vi "Meas Result Generate TWM Digitizer Correction - Generate Files.vi"(8 "error in (no error)":errorcluster, 10 "correction data":T1, 11 "correction root file":path) -> (0 "error out":errorcluster)   [LabVIEW 2020]
uses:
  Meas Results TWM Digitizer Correction Data.ctl
  Meas Results Correction Structuring Mode.ctl
  other/infolib/String.vi
  other/infolib/I64.vi
  other/infolib/2D EXT.vi
  other/infolib/1D EXT.vi
  other/infolib/1D String.vi
  other/infolib/1D I64.vi
  other/infolib/infolib.lvlib
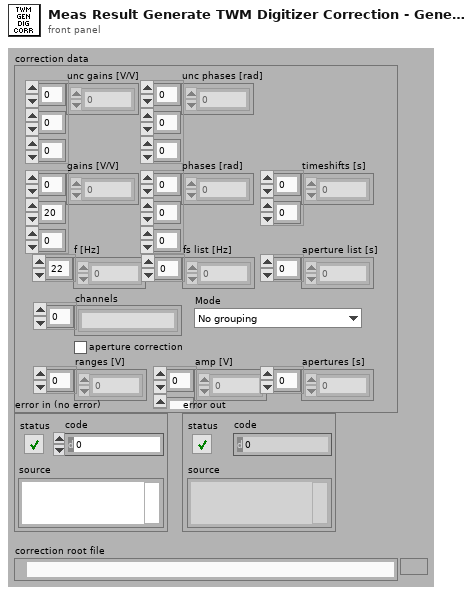
[diagram p1: front panel]
types:
  T1 = typedef "Meas Results TWM Digitizer Correction Data.ctl" = cluster{"gains [V/V]":dbl[][][], "phases [rad]":dbl[][][], "timeshifts [s]":dbl[][], "f [Hz]":dbl[], "fs list [Hz]":dbl[], "aperture list [s]":dbl[], "channels":string[], "Mode":T2, "aperture correction":bool, "ranges [V]":dbl[], "amp [V]":dbl[][], "apertures [s]":dbl[], "unc gains [V/V]":dbl[][][], "unc phases [rad]":dbl[][][]}
  T2 = typedef "Meas Results Correction Structuring Mode.ctl" = enum16{"No grouping", "Group by apertures (3458A)", "Group by fs (generic digitizer)"}
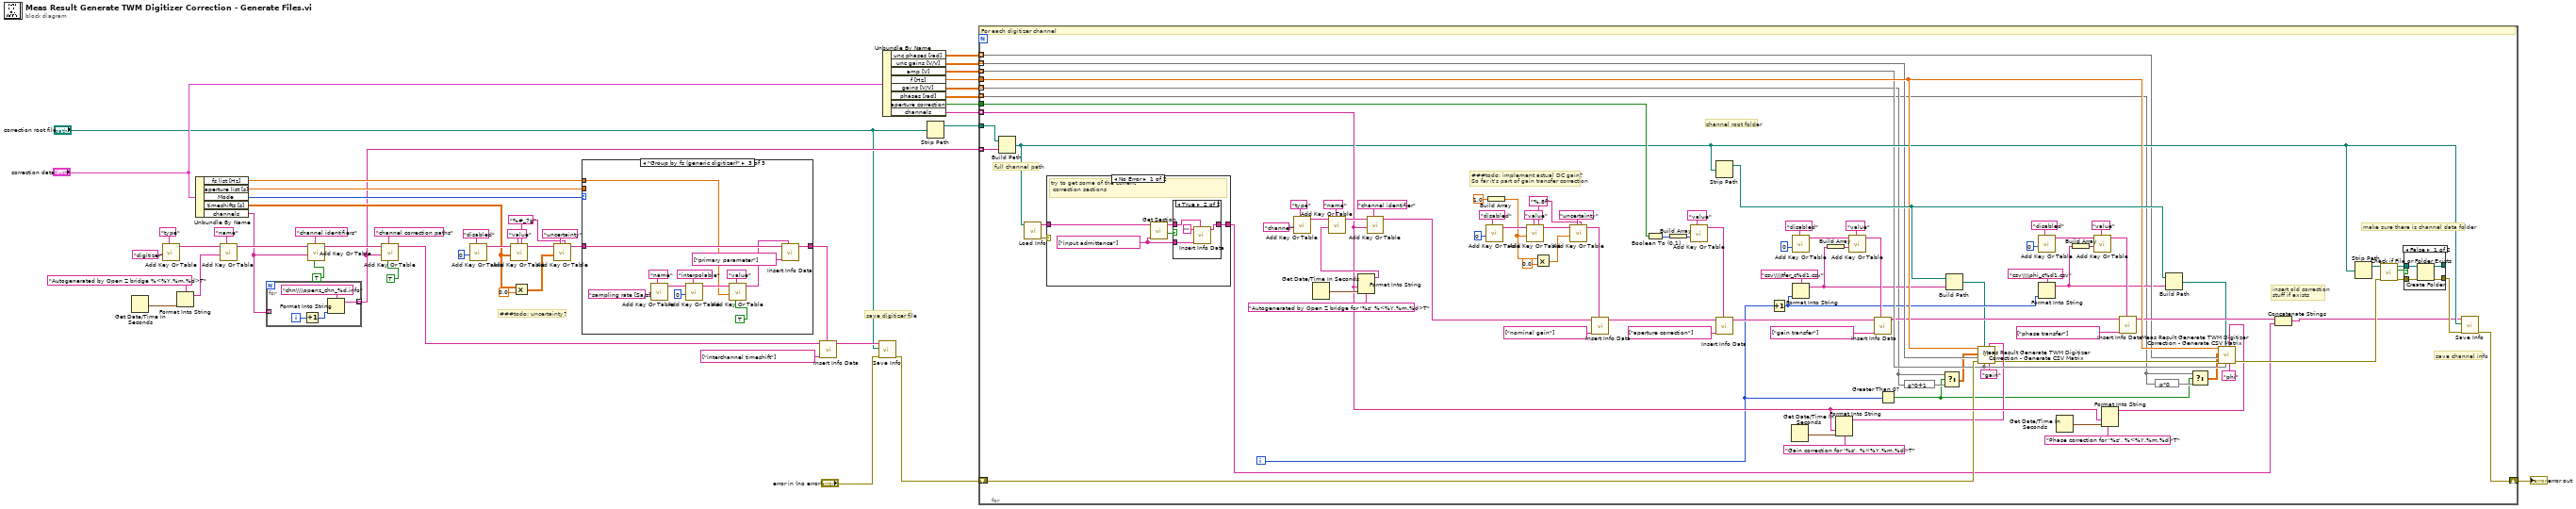
[diagram p0: block diagram]
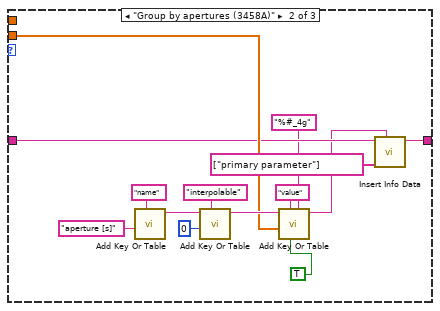
[diagram p6: hidden frame]
diagram:
  w8 = "%#_7g" ("format string (%_20f)")
  # "save digitizer file"
  # "###todo: uncertainty?"
  n1 = Get Date/Time In Seconds() -> (seconds since 1Jan1904=w42:timestamp)
  n2 = call-poly "Add Key Or Table.vi"("key description"="type", "string"="digitizer") -> ("info data out"=w44:string)  [unwired: 8 in, 1 out]
  n3 = Format Into String(format string="Autogenerated by Open Z bridge %<%Y.%m.%d>T", w42) -> (resulting string=w41:string)  [unwired: 2 in, 1 out]
  n4 = Unbundle By Name("correction data") -> ("fs list [Hz]"=w23:dbl[], "aperture list [s]"=w24:dbl[], "Mode"=w25:T2, "timeshifts [s]"=w29:dbl[][], "channels"=w36:string[])
  n5 = call-poly "Add Key Or Table.vi"("key description"="name", "string"=w41, "info data"=w44) -> ("info data out"=w39:string)  [unwired: 7 in, 1 out]
  n6 = for {
    tunnel: w36 -> [_] mode=indexing
    tunnel: [w50] -> w19 mode=indexing
    i -> [w49]
    n7 = Increment(x=w49) -> (x+1=w48:i32)
    n8 = Format Into String(format string="chn\\\\openz_chn_%d.info", w48) -> (resulting string=w50:string)  [unwired: 2 in, 1 out]
  }
  n9 = call-poly "Add Key Or Table.vi"("collumn vector (F)"=TRUE ("column vector (F)"), "key description"="channel identifiers", "string"=w36, "info data"=w39) -> ("info data out"=w37:string)  [unwired: 6 in, 1 out]
  n10 = call-poly "Add Key Or Table.vi"("collumn vector (F)"=TRUE ("column vector (F)"), "key description"="channel correction paths", "string"=w19, "info data"=w37) -> ("info data out"=w21:string)  [unwired: 6 in, 1 out]
  n11 = call-poly "Add Key Or Table.vi"("key description"="disabled", "numeric"=i64 0) -> ("info data out"=w32:string)  [unwired: 8 in, 1 out]
  n12 = call-poly "Add Key Or Table.vi"("format string (%.;%#_20f)"=w8, "key description"="value", "numeric"=w29, "info data"=w32) -> ("info data out"=w30:string)  [unwired: 6 in, 1 out]
  n13 = Multiply(x=w29, y=0.0) -> (x*y=w28:dbl[][])
  n14 = call-poly "Add Key Or Table.vi"("format string (%.;%#_20f)"=w8, "key description"="uncertainty", "numeric"=w28, "info data"=w30) -> ("info data out"=w26:string)  [unwired: 6 in, 1 out]
  n15 = case shown="\"Group by fs (generic digitizer)\"" w25 {
    tunnel: w26 -> [w52 w58 w72]
    tunnel: w24 -> [_ w59 _]
    tunnel: [w52 w55 w69] -> w22
    tunnel: w23 -> [_ _ w68]
    frame "No grouping", Default {
    }
    frame "Group by apertures (3458A)" {
      n16 = call-poly "Add Key Or Table.vi"("key description"="name", "string"="aperture [s]") -> ("info data out"=w63:string)  [unwired: 8 in, 1 out]
      n17 = call-poly "Add Key Or Table.vi"("key description"="interpolable", "numeric"=i64 0, "info data"=w63) -> ("info data out"=w60:string)  [unwired: 7 in, 1 out]
      n18 = call-poly "Add Key Or Table.vi"("format string (%.;%#_20f)"="%#_4g" ("format string (%_20f)"), "collumn vector (F)"=TRUE ("column vector (F)"), "key description"="value", "numeric"=w59, "info data"=w60) -> ("info data out"=w57:string)  [unwired: 5 in, 1 out]
      n19 = call "Insert Info Data.vi"("info data to insert"=w57, "sections"=string[] ["primary parameter"], "info data"=w58) -> ("info data out"=w55:string)  [unwired: 7 in, 1 out]
    }
    frame "Group by fs (generic digitizer)" {
      n20 = call-poly "Add Key Or Table.vi"("key description"="name", "string"="sampling rate [Sa/s]") -> ("info data out"=w76:string)  [unwired: 8 in, 1 out]
      n21 = call-poly "Add Key Or Table.vi"("key description"="interpolable", "numeric"=i64 0, "info data"=w76) -> ("info data out"=w73:string)  [unwired: 7 in, 1 out]
      n22 = call-poly "Add Key Or Table.vi"("collumn vector (F)"=TRUE ("column vector (F)"), "key description"="value", "numeric"=w68, "info data"=w73) -> ("info data out"=w71:string)  [unwired: 6 in, 1 out]
      n23 = call "Insert Info Data.vi"("info data to insert"=w71, "sections"=string[] ["primary parameter"], "info data"=w72) -> ("info data out"=w69:string)  [unwired: 7 in, 1 out]
    }
  }
  n24 = call "Insert Info Data.vi"("info data to insert"=w22, "sections"=string[] ["interchannel timeshift"], "info data"=w21) -> ("info data out"=w15:string)  [unwired: 7 in, 1 out]
  n25 = call "Save Info.vi"("error in"="error in (no error)", "filename"="correction root file", "info data"=w15) -> ("error out"=w13:errorcluster)  [unwired: 8 in]
  n26 = Unbundle By Name("correction data") -> ("unc phases [rad]"=w3:dbl[][][], "unc gains [V/V]"=w4:dbl[][][], "amp [V]"=w5:dbl[][], "f [Hz]"=w9:dbl[], "gains [V/V]"=w7:dbl[][][], "phases [rad]"=w6:dbl[][][], "aperture correction"=w16:bool, "channels"=w17:string[])
  n27 = Strip Path(path="correction root file") -> (stripped path=w12:path)  [unwired: 1 out]
  n28 = for {
    tunnel: w19 -> [w171] mode=indexing
    tunnel: w12 -> [w170]
    tunnel: w17 -> [w133] mode=indexing
    tunnel: w16 -> [w142]
    shift-right: [w135] -> w10
    shift-left: w13 -> [w131]
    tunnel: w6 -> [w81] mode=indexing
    tunnel: w9 -> [w132]
    tunnel: w7 -> [w84] mode=indexing
    tunnel: w5 -> [w121] mode=indexing
    tunnel: w4 -> [w120] mode=indexing
    tunnel: w3 -> [w119] mode=indexing
    i -> [w86]
    w128 = "%.8f" ("format string (%_20f)")
    # "insert old correction\nstuff if exists"
    # "full channel path"
    # "channel root folder"
    # "make sure there is channel data folder"
    # "save channel info"
    # "###todo: implement actual DC gain?\nSo far it's part of gain transfer correction"
    # "For each digitizer channel"
    n29 = Build Path(base path=w170, name or relative path=w171) -> (appended path=w127:path)
    n30 = call "Load Info.vi"("filename"=w127) -> ("error out"=w126:errorcluster, "info data"=w125:string)  [unwired: 9 in]
    n31 = case shown="No Error" w126 {
      tunnel: w125 -> [w176 _]
      tunnel: [w173 _] -> w122
      frame No Error {
        w172 = string[] ["input admittance"] ("sections")
        # "try to get some of the current\n correction sections"
        n32 = call "Get Section.vi"("sections"=w172, "info data"=w176) -> ("exist"=w175:bool, "section part"=w174:string)  [unwired: 7 in, 1 out]
        n33 = case shown="True" w175 {
          tunnel: w174 -> [_ w178]
          tunnel: w172 -> [_ w180]
          tunnel: [_ w179] -> w173
          frame False {
          }
          frame True {
            n34 = call "Insert Info Data.vi"("info data to insert"=w178, "sections"=w180, "info data"="") -> ("info data out"=w179:string)  [unwired: 7 in, 1 out]
          }
        }
      }
      frame Error {
      }
    }
    n35 = call-poly "Add Key Or Table.vi"("key description"="type", "string"="channel") -> ("info data out"=w167:string)  [unwired: 8 in, 1 out]
    n36 = Get Date/Time In Seconds() -> (seconds since 1Jan1904=w163:timestamp)
    n37 = Format Into String(format string="Autogenerated by Open Z bridge for '%s' %<%Y.%m.%d>T", w133, w163) -> (resulting string=w161:string)  [unwired: 2 in, 1 out]
    n38 = call-poly "Add Key Or Table.vi"("key description"="name", "string"=w161, "info data"=w167) -> ("info data out"=w169:string)  [unwired: 7 in, 1 out]
    n39 = call-poly "Add Key Or Table.vi"("key description"="channel identifier", "string"=w133, "info data"=w169) -> ("info data out"=w149:string)  [unwired: 7 in, 1 out]
    n40 = call-poly "Add Key Or Table.vi"("key description"="disabled", "numeric"=i64 0) -> ("info data out"=w158:string)  [unwired: 8 in, 1 out]
    n41 = Build Array(1.0) -> (w152:dbl[])
    n42 = call-poly "Add Key Or Table.vi"("format string (%.;%#_20f)"=w128, "key description"="value", "numeric"=w152, "info data"=w158) -> ("info data out"=w160:string)  [unwired: 6 in, 1 out]
    n43 = Multiply(x=w152, y=0.0) -> (x*y=w153:dbl[])
    n44 = call-poly "Add Key Or Table.vi"("format string (%.;%#_20f)"=w128, "key description"="uncertainty", "numeric"=w153, "info data"=w160) -> ("info data out"=w150:string)  [unwired: 6 in, 1 out]
    n45 = call "Insert Info Data.vi"("info data to insert"=w150, "sections"=string[] ["nominal gain"], "info data"=w149) -> ("info data out"=w145:string)  [unwired: 7 in, 1 out]
    n46 = Boolean To (0,1)(Boolean=w142) -> (0, 1=w143:i16)
    n47 = Build Array(w143) -> (w129:i16[])
    n48 = call-poly "Add Key Or Table.vi"("key description"="value", "numeric"=w129) -> ("info data out"=w144:string)  [unwired: 8 in, 1 out]
    n49 = Strip Path(path=w127) -> (stripped path=w134:path)  [unwired: 1 out]
    n50 = call "Insert Info Data.vi"("info data to insert"=w144, "sections"=string[] ["aperture correction"], "info data"=w145) -> ("info data out"=w141:string)  [unwired: 7 in, 1 out]
    n51 = Increment(x=w86) -> (x+1=w101:i32)
    n52 = Get Date/Time In Seconds() -> (seconds since 1Jan1904=w98:timestamp)
    n53 = call-poly "Add Key Or Table.vi"("key description"="disabled", "numeric"=i64 0) -> ("info data out"=w115:string)  [unwired: 8 in, 1 out]
    n54 = Format Into String(format string="csv\\\\tfer_c%d1.csv", w101) -> (resulting string=w100:string)  [unwired: 2 in, 1 out]
    n55 = Build Array(w100) -> (w111:string[])
    n56 = Format Into String(format string="Gain correction for '%s', %<%Y.%m.%d>T", w133, w98) -> (resulting string=w96:string)  [unwired: 2 in, 1 out]
    n57 = call-poly "Add Key Or Table.vi"("key description"="value", "string"=w111, "info data"=w115) -> ("info data out"=w113:string)  [unwired: 7 in, 1 out]
    n58 = call "Insert Info Data.vi"("info data to insert"=w113, "sections"=string[] ["gain transfer"], "info data"=w141) -> ("info data out"=w102:string)  [unwired: 7 in, 1 out]
    n59 = Greater Than 0?(x=w86) -> (x > 0?=w80:bool)
    n60 = expression code="g*0+1"(w84) -> (w85:dbl[][])
    n61 = Select(t=w84, s=w80, f=w85) -> (s? t:f=w87:dbl[][])
    n62 = Build Path(base path=w134, name or relative path=w100) -> (appended path=w99:path)
    n63 = call "Meas Result Generate TWM Digitizer Correction - Generate CSV Matrix.vi"("header"="gain", "comment"=w96, "amp [V]"=w121, "CSV path"=w99, "error in (no error)"=w131, "uncertainty"=w120, "data"=w87, "f [Hz]"=w132) -> ("error out"=w91:errorcluster)  [unwired: 3 in]
    n64 = call-poly "Add Key Or Table.vi"("key description"="disabled", "numeric"=i64 0) -> ("info data out"=w106:string)  [unwired: 8 in, 1 out]
    n65 = Format Into String(format string="csv\\\\phi_c%d1.csv", w101) -> (resulting string=w92:string)  [unwired: 2 in, 1 out]
    n66 = Get Date/Time In Seconds() -> (seconds since 1Jan1904=w93:timestamp)
    n67 = Build Array(w92) -> (w110:string[])
    n68 = call-poly "Add Key Or Table.vi"("key description"="value", "string"=w110, "info data"=w106) -> ("info data out"=w108:string)  [unwired: 7 in, 1 out]
    n69 = Format Into String(format string="Phase correction for '%s', %<%Y.%m.%d>T", w133, w93) -> (resulting string=w95:string)  [unwired: 2 in, 1 out]
    n70 = call "Insert Info Data.vi"("info data to insert"=w108, "sections"=string[] ["phase transfer"], "info data"=w102) -> ("info data out"=w124:string)  [unwired: 7 in, 1 out]
    n71 = expression code="p*0"(w81) -> (w83:dbl[][])
    n72 = Build Path(base path=w134, name or relative path=w92) -> (appended path=w90:path)
    n73 = Select(t=w81, s=w80, f=w83) -> (s? t:f=w82:dbl[][])
    n74 = call "Meas Result Generate TWM Digitizer Correction - Generate CSV Matrix.vi"("header"="phi", "comment"=w95, "amp [V]"=w121, "CSV path"=w90, "error in (no error)"=w91, "uncertainty"=w119, "data"=w82, "f [Hz]"=w132) -> ("error out"=w130:errorcluster)  [unwired: 3 in]
    n75 = Concatenate Strings(w124, w122) -> (w123:string)
    n76 = Strip Path(path=w127) -> (stripped path=w140:path)  [unwired: 1 out]
    n77 = call <vilib>:"Check if File or Folder Exists.vi"("error in (no error)"=w130, "path"=w140) -> ("error out"=w137:errorcluster, "file or folder exists?"=w139:bool, "dup path"=w138:path)  [unwired: 7 in]
    n78 = case shown="False" w139 {
      tunnel: w138 -> [w184 w185]
      tunnel: [w183 w185] -> _
      tunnel: w137 -> [w182 w186]
      tunnel: [w181 w186] -> w136
      frame False {
        n79 = Create Folder(path (use dialog)=w184, error in=w182) -> (created path=w183:path, error out=w181:errorcluster)  [unwired: 1 in, 1 out]
      }
      frame True {
      }
    }
    n80 = call "Save Info.vi"("error in"=w136, "filename"=w127, "info data"=w123) -> ("error out"=w135:errorcluster)  [unwired: 8 in]
  }
  "error out" <- w10
